vi "副屏设置.vi"() -> ()   [LabVIEW 2016, in "副屏.lvlib"]
uses:
  <vilib>/Utility/config.llb/NI_LVConfig.lvlib
panel:
  in  "关闭":bool
  in  "底部状态栏显示信息":string="一体化微型水质监测系统"
  in  "流速":bool caption="氨氮禁用"
  in  "瞬时流量":bool caption="氨氮禁用"
  in  "湿度":bool=TRUE caption="氨氮禁用"
  in  "水位":bool caption="氨氮禁用"
  in  "室温":bool=TRUE caption="氨氮禁用"
  in  "CODCr":bool caption="氨氮禁用"
  in  "CODMn":bool caption="氨氮禁用"
  in  "总氮":bool caption="氨氮禁用"
  in  "总磷":bool caption="氨氮禁用"
  in  "氨氮":bool caption="氨氮禁用"
  in  "Turb":bool caption="氨氮禁用"
  in  "Cond":bool caption="氨氮禁用"
  in  "DO":bool caption="氨氮禁用"
  in  "pH":bool caption="氨氮禁用"
  in  "水温":bool caption="氨氮禁用"
  # "副屏显示信息设置"
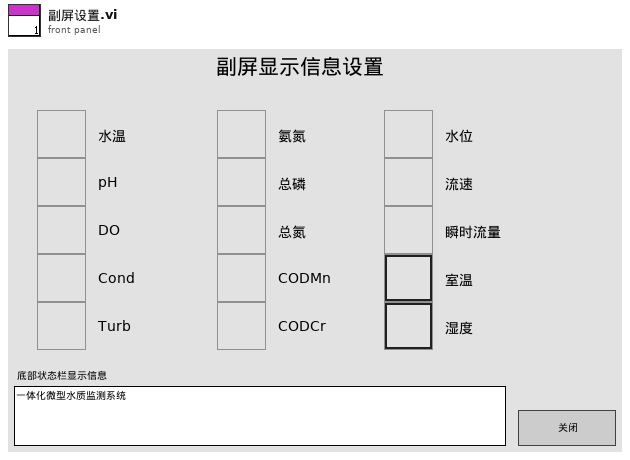
[diagram p1: front panel]
types:
  T1 = typedef "NI_LVConfig.lvlib/Config Data RefNum.ctl" = refnum<k1>
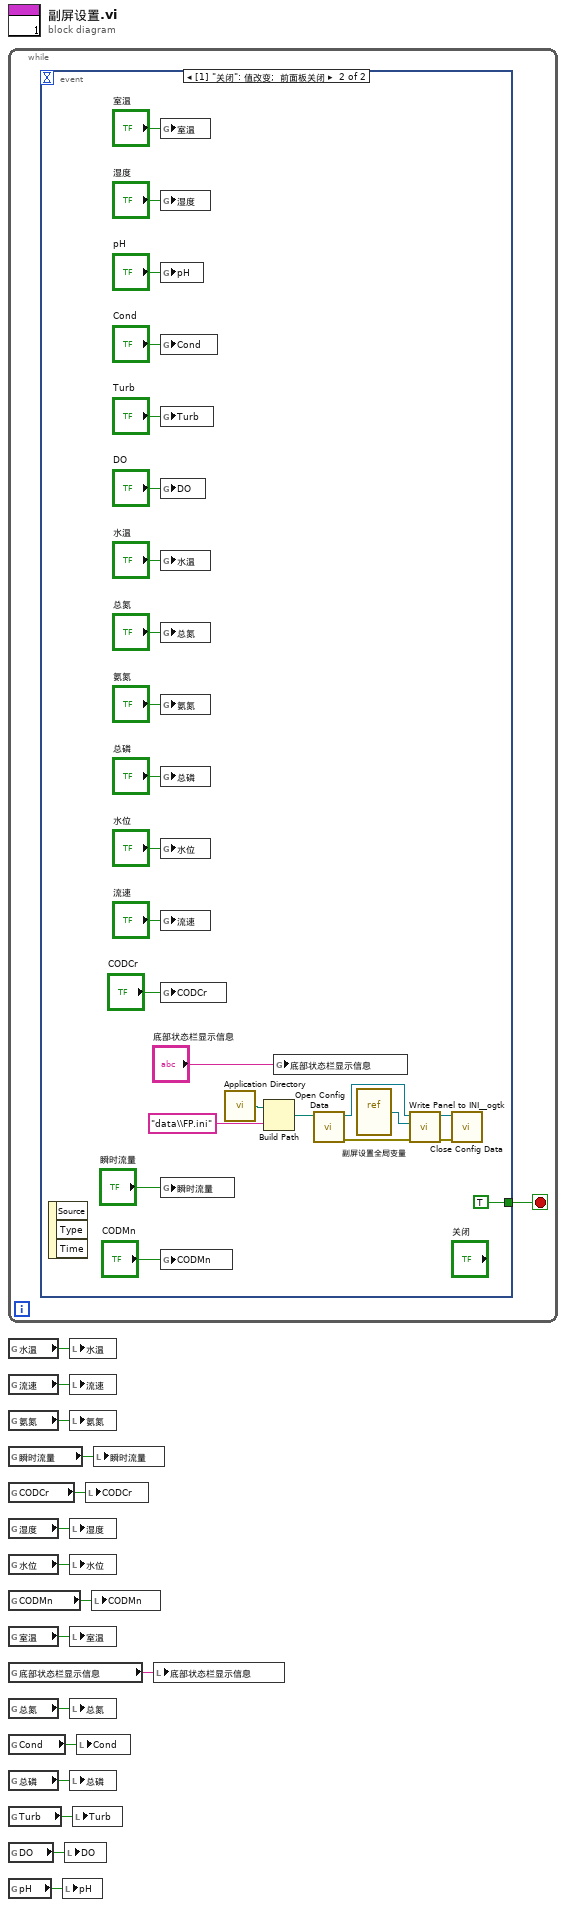
[diagram p0: block diagram]
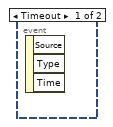
[diagram p2: hidden frame]
diagram:
  n1 = while {
    stop <- w17 stop-if-true
    n2 = event shown="[1] \"关闭\": 值改变;  前面板关闭" {
      selector: _ -> [_ _]
      dyn-events: _ -> [_ _]
      timeout: _ -> [_ _]
      tunnel: [_ TRUE] -> w17
      event Timeout {
        n3 = event-data() -> ()  [unwired: 1 in, 3 out]
      }
      event "关闭": Value Change; Panel Close {
        n4 = event-data() -> ()  [unwired: 1 in, 3 out]
        n5 = global write "副屏设置全局变量.vi" "室温"("室温") -> ()
        n6 = global write "副屏设置全局变量.vi" "湿度"("湿度") -> ()
        n7 = global write "副屏设置全局变量.vi" "pH"("pH") -> ()
        n8 = global write "副屏设置全局变量.vi" "Cond"("Cond") -> ()
        n9 = global write "副屏设置全局变量.vi" "Turb"("Turb") -> ()
        n10 = global write "副屏设置全局变量.vi" "DO"("DO") -> ()
        n11 = global write "副屏设置全局变量.vi" "水温"("水温") -> ()
        n12 = global write "副屏设置全局变量.vi" "总氮"("总氮") -> ()
        n13 = global write "副屏设置全局变量.vi" "氨氮"("氨氮") -> ()
        n14 = global write "副屏设置全局变量.vi" "总磷"("总磷") -> ()
        n15 = global write "副屏设置全局变量.vi" "水位"("水位") -> ()
        n16 = global write "副屏设置全局变量.vi" "流速"("流速") -> ()
        n17 = global write "副屏设置全局变量.vi" "CODCr"("CODCr") -> ()
        n18 = global write "副屏设置全局变量.vi" "瞬时流量"("瞬时流量") -> ()
        n19 = global write "副屏设置全局变量.vi" "CODMn"("CODMn") -> ()
        n20 = call <vilib>:"Application Directory.vi"() -> ("Application Directory"=w41:path)
        n21 = Build Path(base path=w41, name or relative path="data\\FP.ini" ("名称或相对路径")) -> (appended path=w39:path)
        n22 = global write "副屏设置全局变量.vi" "底部状态栏显示信息"("底部状态栏显示信息") -> ()
        n23 = call <vilib>:"Open Config Data.vi"("configuration file path"=w39) -> ("error out"=w35:errorcluster, "refnum"=w38:T1)  [unwired: 8 in, 1 out]
        n24 = vi-ref "副屏设置全局变量.vi"() -> (w37:refnum<vi>)
        n25 = call <userlib>:"Write Panel to INI__ogtk.vi"("error in (no error)"=w35, "VI ref"=w37, "refnum"=w38) -> ("error out"=w34:errorcluster, "refnum out"=w36:T1)  [unwired: 7 in]
        n26 = call <vilib>:"Close Config Data.vi"("error in (no error)"=w34, "refnum"=w36) -> ()  [unwired: 8 in, 2 out]
      }
    }
  }
  n27 = global read "副屏设置全局变量.vi" "水温"() -> (w16:bool)
  n28 = global read "副屏设置全局变量.vi" "流速"() -> (w10:bool)
  n29 = global read "副屏设置全局变量.vi" "氨氮"() -> (w15:bool)
  n30 = global read "副屏设置全局变量.vi" "瞬时流量"() -> (w8:bool)
  n31 = global read "副屏设置全局变量.vi" "CODCr"() -> (w14:bool)
  n32 = global read "副屏设置全局变量.vi" "湿度"() -> (w7:bool)
  n33 = global read "副屏设置全局变量.vi" "水位"() -> (w13:bool)
  n34 = global read "副屏设置全局变量.vi" "CODMn"() -> (w12:bool)
  n35 = global read "副屏设置全局变量.vi" "室温"() -> (w4:bool)
  n36 = global read "副屏设置全局变量.vi" "底部状态栏显示信息"() -> (w11:string)
  n37 = global read "副屏设置全局变量.vi" "总氮"() -> (w5:bool)
  n38 = global read "副屏设置全局变量.vi" "Cond"() -> (w9:bool)
  n39 = global read "副屏设置全局变量.vi" "总磷"() -> (w2:bool)
  n40 = global read "副屏设置全局变量.vi" "Turb"() -> (w3:bool)
  n41 = global read "副屏设置全局变量.vi" "DO"() -> (w6:bool)
  n42 = global read "副屏设置全局变量.vi" "pH"() -> (w1:bool)
  n43 = local write "pH"(w1) -> ()
  n44 = local write "DO"(w6) -> ()
  n45 = local write "水温"(w16) -> ()
  n46 = local write "流速"(w10) -> ()
  n47 = local write "氨氮"(w15) -> ()
  n48 = local write "湿度"(w7) -> ()
  n49 = local write "水位"(w13) -> ()
  n50 = local write "室温"(w4) -> ()
  n51 = local write "总氮"(w5) -> ()
  n52 = local write "总磷"(w2) -> ()
  n53 = local write "Turb"(w3) -> ()
  n54 = local write "Cond"(w9) -> ()
  n55 = local write "CODCr"(w14) -> ()
  n56 = local write "CODMn"(w12) -> ()
  n57 = local write "瞬时流量"(w8) -> ()
  n58 = local write "底部状态栏显示信息"(w11) -> ()
